vi "RDS Child Receive Message.vi"(8 "error in (no error)":errorcluster, 10 "RDS Message":refnum<class "RDS Message.lvclass">, 11 "RDS Logger Actor in":refnum<class "RDS Logger Actor.lvclass">) -> (0 "error out":errorcluster, 3 "RDS Logger Actor out":refnum<class "RDS Logger Actor.lvclass">)   [LabVIEW 2015, in "RDS Logger Actor.lvlib" / "RDS Logger Actor.lvclass"]
uses:
  RDS Logger Actor.lvclass
  Libraries/RDS Framework/RDS Message Class/RDS Message.lvclass
  Libraries/RDS Framework/RDS Message Class/RDS Message.lvclass/RDS Message.ctl
  Libraries/RDS Child Messages/State Sample Message/State Sample Message.lvclass
  Libraries/RDS Child Messages/State Sample Message/State Sample Message.lvclass/State Sample Message.ctl
  RDS Logger Actor.lvclass/RDS Logger Actor.ctl
  RDS State Tracker/RDS State/RDS State.lvclass
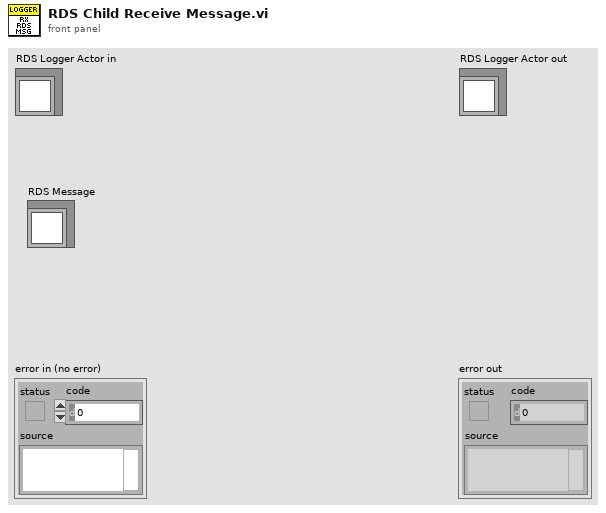
[diagram p1: front panel]
types:
  T1 = typedef "RDS Child Messages.lvlib/RDS Message ID.ctl" = enum16{"RDS Hello World", "String Message", "AIP_Status", "AIP_Command", "GPS_Data", "MCB_Command", "MCB_Status", "Compass_Data", "Depth_Data", "Battery_Data", "Contoller_State", "Set_Mag_Dev", "BTB_Shutdown", "State_Sample_Request", "State_Sample", "PID_Gains_Set", "Helm_Limiter_Set", "Helm_Heading_Command", "Helm_Steering_Command", "Helm_Status", "Controller_Message", "AIP_Set_Min_Depth", "Mission_Controller_State", "Mission_Upload", "Mission_Set_Op_and_Run", "Mission_Settings_Set"}
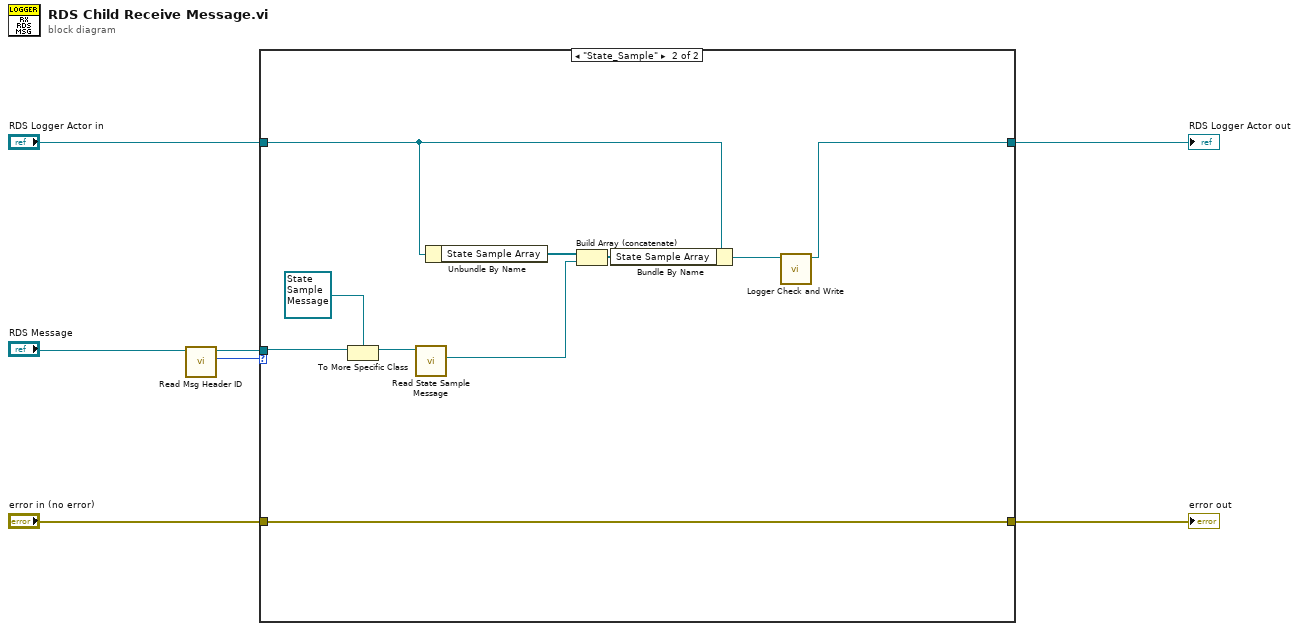
[diagram p0: block diagram]
diagram:
  n1 = call "Read Msg Header ID.vi"("RDS Message in"="RDS Message") -> ("Msg ID"=w6:T1, "RDS Message out"=w2:refnum<class "RDS Message.lvclass">)  [unwired: 6 in, 3 out]
  n2 = case shown="\"State_Sample\"" w6 {
    tunnel: "RDS Logger Actor in" -> [w8 w12]
    tunnel: [w9 w19] -> w4
    tunnel: "error in (no error)" -> [w9 w19]
    tunnel: w2 -> [_ w18]
    tunnel: [w8 w10] -> w1
    frame "RDS Hello World", Default {
    }
    frame "State_Sample" {
      n3 = To More Specific Class(target class=refnum<class "State Sample Message.lvclass"> refnum ("RDS Child Messages.lvlib:State Sample Message.lvclass"), reference=w18) -> (specific class reference=w15:refnum<class "State Sample Message.lvclass">)  [unwired: 1 in, 1 out]
      n4 = call "Read State Sample Message.vi"("State Sample Message in"=w15) -> ("State Sample"=w14:refnum<class "RDS State.lvclass">)  [unwired: 8 in, 2 out]
      n5 = Unbundle By Name(w12) -> ("State Sample Array"=w16:refnum<class "RDS State.lvclass">[])
      n6 = Build Array (concatenate)(w16, w14) -> (w13:refnum<class "RDS State.lvclass">[])
      n7 = Bundle By Name(cluster=w12, "State Sample Array"=w13) -> (w11:refnum<class "RDS Logger Actor.lvclass">)
      n8 = call "Logger Check and Write.vi"("RDS Logger Actor in"=w11) -> ("RDS Logger Actor out"=w10:refnum<class "RDS Logger Actor.lvclass">)  [unwired: 9 in, 1 out]
    }
  }
  "error out" <- w4
  "RDS Logger Actor out" <- w1
